vi "Set State Value.vi"(8 "error in":errorcluster, 9 "value":i32, 10 "state":string, 11 "routing channel in":T1 format="%.0x") -> (0 "error out":errorcluster, 3 "routing channel out":T1=18446744073709551615 format="%.0x")   [LabVIEW 2020, in "Routing and Faulting Scripting.lvlib"]
doc: "Sets the numeric value of the state."
uses:
  Routing and Faulting Scripting.lvlib
  <vilib>/NI VeriStand/Custom Device API/Custom Device Item Ref.ctl
  <vilib>/NI VeriStand/Custom Device API/Custom Device API.lvlib
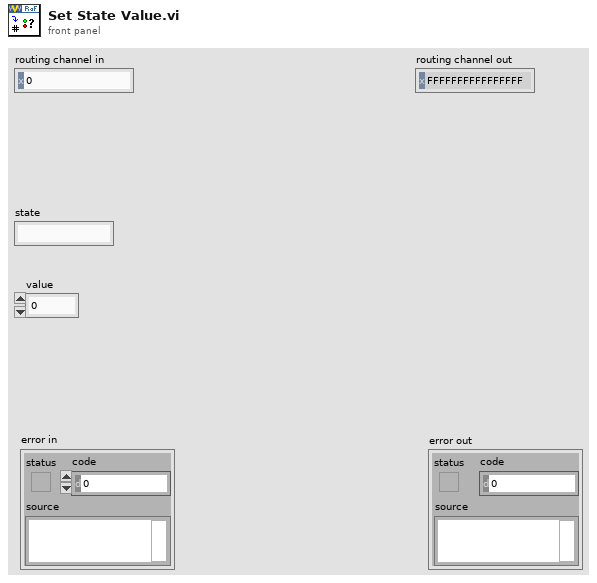
[diagram p1: front panel]
types:
  T1 = typedef "Custom Device API.lvlib/Custom Device Item Ref.ctl" = u64
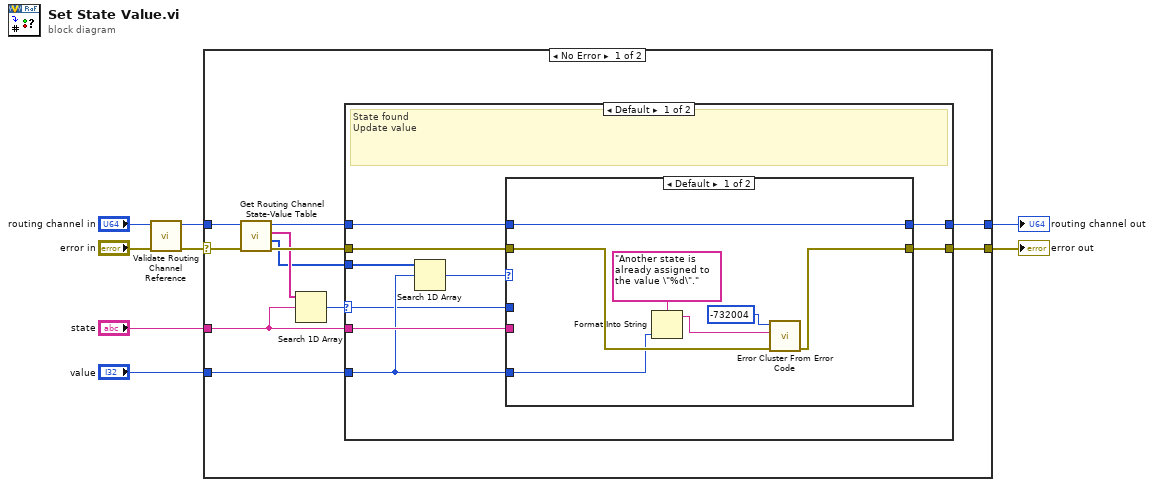
[diagram p0: block diagram]
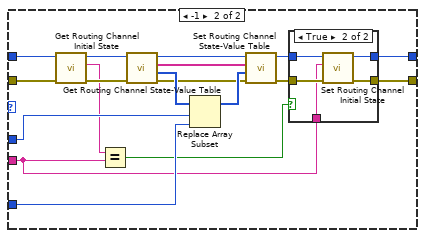
[diagram p2: hidden frame]
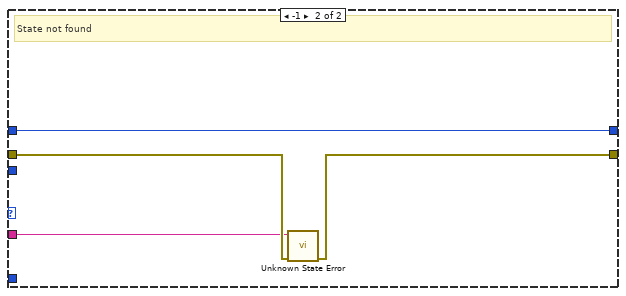
[diagram p4: hidden frame]
diagram:
  n1 = call "Validate Routing Channel Reference.vi"("error in"="error in", "routing channel in"="routing channel in") -> ("error out"=w3:errorcluster, "routing channel out"=w1:T1)  [unwired: 8 in]
  n2 = case shown="No Error" w3 {
    selector: w3 -> [w19 w66]
    tunnel: [w15 w66] -> w4
    tunnel: [w16 w65] -> w5
    tunnel: "state" -> [w13 _]
    tunnel: "value" -> [w10 _]
    tunnel: w1 -> [w9 w65]
    frame No Error {
      n3 = call "Get Routing Channel State-Value Table.vi"("error in"=w19, "routing channel in"=w9) -> ("error out"=w17:errorcluster, "state values"=w12:i32[], "state names"=w14:string[], "routing channel out"=w18:T1)  [unwired: 6 in]
      n4 = Search 1D Array(1D array=w14, element=w13) -> (index of element=w11:i32)  [unwired: 1 in]
      n5 = case shown="Default" w11 {
        selector: w11 -> [w20 _]
        tunnel: w18 -> [w28 w62]
        tunnel: w17 -> [w27 w64]
        tunnel: w12 -> [w22 _]
        tunnel: [w23 w62] -> w16
        tunnel: [w25 w63] -> w15
        tunnel: w13 -> [w26 w61]
        tunnel: w10 -> [w21 _]
        frame Default {
          # "State found\nUpdate value"
          n6 = Search 1D Array(1D array=w22, element=w21) -> (index of element=w24:i32)  [unwired: 1 in]
          n7 = case shown="Default" w24 {
            tunnel: w28 -> [w32 w44]
            tunnel: w27 -> [w34 w45]
            tunnel: w26 -> [_ w37]
            tunnel: [w33 w40] -> w25
            tunnel: [w32 w38] -> w23
            tunnel: w21 -> [w30 w51]
            tunnel: w20 -> [_ w52]
            frame Default {
              n8 = Format Into String(format string="Another state is already assigned to the value \"%d\"." ("error message (\"\")"), w30) -> (resulting string=w29:string)  [unwired: 2 in, 1 out]
              n9 = call <vilib>:"Error Cluster From Error Code.vi"("error in (no error)"=w34, "error message (\"\")"=w29, "error code (0)"=-732004) -> ("error out"=w33:errorcluster)  [unwired: 6 in]
            }
            frame -1 {
              n10 = call "Get Routing Channel Initial State.vi"("error in"=w45, "routing channel in"=w44) -> ("error out"=w42:errorcluster, "initial state"=w41:string, "routing channel out"=w43:T1)  [unwired: 7 in]
              n11 = Equal?(x=w41, y=w37) -> (x = y?=w36:bool)
              n12 = call "Get Routing Channel State-Value Table.vi"("error in"=w42, "routing channel in"=w43) -> ("error out"=w47:errorcluster, "state values"=w53:i32[], "state names"=w49:string[], "routing channel out"=w48:T1)  [unwired: 6 in]
              n13 = Replace Array Subset(array=w53, new element=w51, index=w52) -> (w50:i32[])
              n14 = call "Set Routing Channel State-Value Table.vi"("error in"=w47, "state values"=w50, "state names"=w49, "routing channel in"=w48) -> ("error out"=w46:errorcluster, "routing channel out"=w39:T1)  [unwired: 6 in]
              n15 = case shown="True" w36 {
                tunnel: w46 -> [w54 w60]
                tunnel: [w54 w59] -> w40
                tunnel: w39 -> [w55 w58]
                tunnel: [w55 w57] -> w38
                tunnel: w37 -> [_ w56]
                frame False {
                }
                frame True {
                  n16 = call "Set Routing Channel Initial State.vi"("error in"=w60, "state"=w56, "routing channel in"=w58) -> ("error out"=w59:errorcluster, "routing channel out"=w57:T1)  [unwired: 7 in]
                }
              }
            }
          }
        }
        frame -1 {
          # "State not found"
          n17 = call "Unknown State Error.vi"("error in (no error)"=w64, "state"=w61) -> ("error out"=w63:errorcluster)  [unwired: 9 in]
        }
      }
    }
    frame Error {
    }
  }
  "routing channel out" <- w5
  "error out" <- w4
